vi "Drive Set autonomous.vi"(8 "error in (no error)":errorcluster, 10 "Y value":dbl, 11 "X value":dbl) -> (0 "error out (no error)":errorcluster)   [LabVIEW 2013]
uses:
  Drive/Drive Global Data.vi
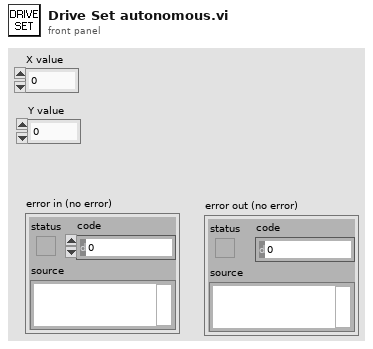
[diagram p1: front panel]
types:
  T1 = cluster{"Y":dbl, "X":dbl, "Left Encoder":dbl, "Right Encoder":dbl, "Slow Drive":bool}
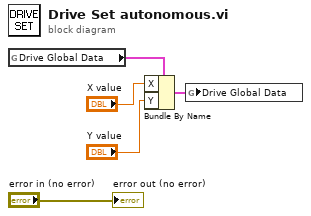
[diagram p0: block diagram]
diagram:
  n1 = global read "Drive Global Data.vi" "Drive Global Data"() -> (w2:T1)
  n2 = Bundle By Name(cluster=w2, "X"="X value", "Y"="Y value") -> (w3:T1)
  n3 = global write "Drive Global Data.vi" "Drive Global Data"(w3) -> ()
  "error out (no error)" <- "error in (no error)"
